vi "Unpack Publish Request.vi"(11 "PublishRequest In":refnum<class "PublishRequest.lvclass">) -> (0 "Publisher ID":string, 1 "Publication Time":timestamp, 2 "Value":variant, 3 "Datum Name":string)   [LabVIEW 2017, in "IMediator.lvlib" / "PublishRequest.lvclass"]
uses:
  PublishRequest.lvclass
  PublishRequest.lvclass/PublishRequest.ctl
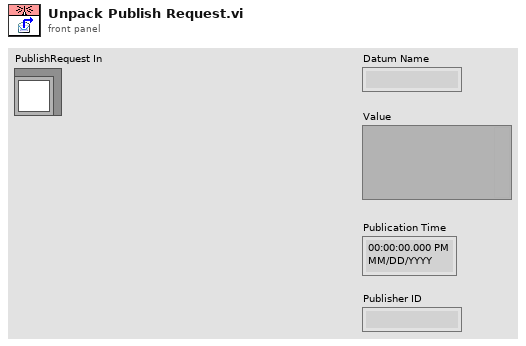
[diagram p1: front panel]
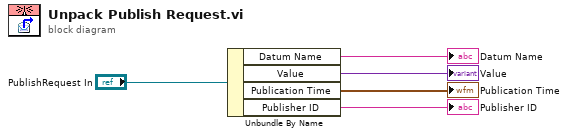
[diagram p0: block diagram]
diagram:
  n1 = Unbundle By Name("PublishRequest In") -> ("Datum Name"=→"Datum Name":string, "Value"=→"Value":variant, "Publication Time"=→"Publication Time":timestamp, "Publisher ID"=→"Publisher ID":string)
